vi "Quick Start - Deadband Simulator.vi"(1 "deadband (%)":dbl=1.0 format="%.2f", 3 "requested pos. (%)":dbl format="%.2f") -> (0 "actual pos. (%)":dbl format="%.2f")   [LabVIEW 2020]
doc: "Deadband generator for simulation. Output won't change until input is at least Deadband percent higher or lower."
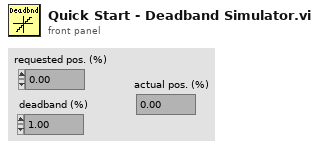
[diagram p1: front panel]
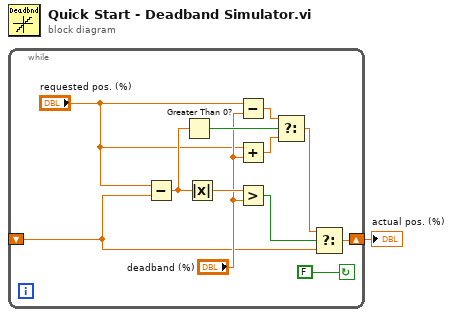
[diagram p0: block diagram]
diagram:
  n1 = while {
    shift-left: _ -> [w4]
    shift-right: [w11] -> w1
    stop <- FALSE continue-if-true
    n2 = Subtract(x="requested pos. (%)", y=w4) -> (x-y=w10:dbl)
    n3 = Greater Than 0?(x=w10) -> (x > 0?=w9:bool)
    n4 = Absolute Value(x=w10) -> (abs(x)=w13:dbl)
    n5 = Subtract(x="requested pos. (%)", y="deadband (%)") -> (x-y=w5:dbl)
    n6 = Add(x="requested pos. (%)", y="deadband (%)") -> (x+y=w6:dbl)
    n7 = Greater?(x=w13, y="deadband (%)") -> (0:w12:bool)
    n8 = Select(t=w5, s=w9, f=w6) -> (s? t:f=w3:dbl)
    n9 = Select(t=w3, s=w12, f=w4) -> (s? t:f=w11:dbl)
  }
  "actual pos. (%)" <- w1
